vi "calibrate steering.vi"(9 "Flip direction?":bool, 10 "Steer motor port":T1=1 items=["Port A", "Port B", "Port C"], 11 "NXT":T2={"error"={"status"=FALSE, "code"=0, "source"=""}, "address"="", "NXT #"=-1, "Show Error"=TRUE, "Connection"=4} {"Connection" items=["USB", "Bluetooth", "USB then Bluetooth", "Last Connection", "Preference"]}) -> (1 "Full right":i16, 2 "Full left":i16, 3 "NXT 2":T2={"error"={"status"=FALSE, "code"=0, "source"=""}, "address"="", "NXT #"=-1, "Show Error"=TRUE, "Connection"=4} caption="NXT" {"Connection" items=["USB", "Bluetooth", "USB then Bluetooth", "Last Connection", "Preference"]})   [LabVIEW 2009]
uses:
  <vilib>/NXT/Subs/LVHSConnector.ctl
  <vilib>/NXT/Block Support/NXT_OutputPort.ctl
  <vilib>/NXT/Dual Mode Library/Motors/MotorDistance_Single.vi
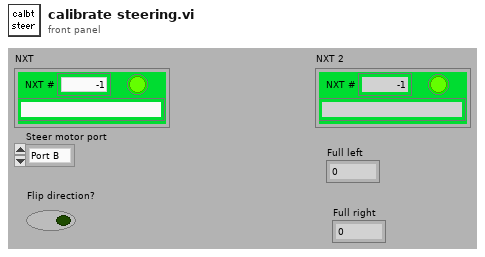
[diagram p1: front panel]
types:
  T1 = typedef "NXT_OutputPort.ctl" = u8
  T2 = typedef "LVHSConnector.ctl" = cluster{"error":errorcluster, "address":string, "NXT #":i32, "Show Error":bool, "Connection":u16}
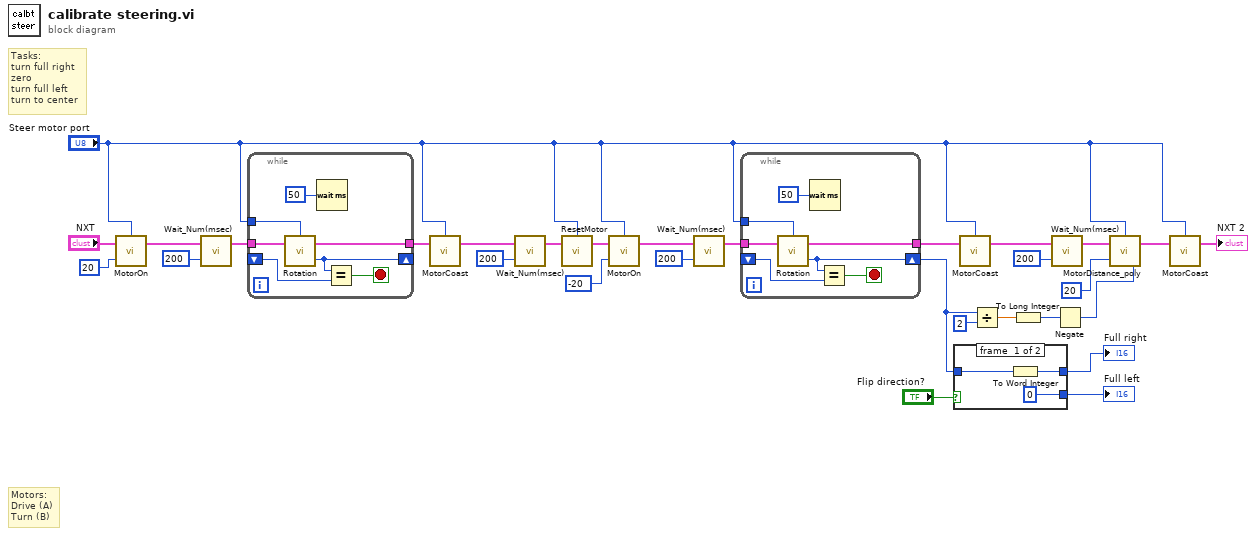
[diagram p0: block diagram]
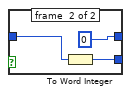
[diagram p2: hidden frame]
diagram:
  # "Motors:\nDrive (A)\nTurn (B)"
  # "Tasks:\nturn full right\nzero\nturn full left\nturn to center"
  n1 = call <vilib>:"MotorOn.vi"("Power (75)"=i8 20, "NXT"="NXT", "Output Port (All Ports)"="Steer motor port") -> ("NXT"=w6:T2)  [unwired: 1 in]
  n2 = call <vilib>:"Wait_Num(msec).vi"("Time (100 msec)"=u32 200 ("Time (msec)"), "NXT"=w6) -> ("NXT"=w5:T2)  [unwired: 2 in]
  n3 = while {
    tunnel: "Steer motor port" -> [w37]
    tunnel: w5 -> [w36]
    tunnel: [w35] -> w29
    shift-right: [w34] -> _
    shift-left: _ -> [w32]
    stop <- w33 stop-if-true
    n4 = call <vilib>:"Rotation.vi"("NXT"=w36, "Port (Port A)"=w37) -> ("Rotation"=w34:i32, "NXT"=w35:T2)  [unwired: 1 in]
    n5 = Wait (ms)(milliseconds to wait=u32 50) -> ()  [unwired: 1 out]
    n6 = Equal?(x=w34, y=w32) -> (x = y?=w33:bool)
  }
  n7 = call <vilib>:"MotorCoast.vi"("NXT"=w29, "Port (All Ports)"="Steer motor port") -> ("NXT"=w15:T2)  [unwired: 2 in]
  n8 = call <vilib>:"Wait_Num(msec).vi"("Time (100 msec)"=u32 200 ("Time (msec)"), "NXT"=w15) -> ("NXT"=w16:T2)  [unwired: 2 in]
  n9 = call <vilib>:"ResetMotor.vi"("NXT"=w16, "Port (All Ports)"="Steer motor port") -> ("NXT"=w27:T2)  [unwired: 2 in]
  n10 = call <vilib>:"MotorOn.vi"("Power (75)"=i8 -20, "NXT"=w27, "Output Port (All Ports)"="Steer motor port") -> ("NXT"=w13:T2)  [unwired: 1 in]
  n11 = call <vilib>:"Wait_Num(msec).vi"("Time (100 msec)"=u32 200 ("Time (msec)"), "NXT"=w13) -> ("NXT"=w14:T2)  [unwired: 2 in]
  n12 = while {
    tunnel: "Steer motor port" -> [w44]
    tunnel: w14 -> [w43]
    tunnel: [w42] -> w22
    shift-right: [w41] -> w3
    shift-left: _ -> [w39]
    stop <- w40 stop-if-true
    n13 = call <vilib>:"Rotation.vi"("NXT"=w43, "Port (Port A)"=w44) -> ("Rotation"=w41:i32, "NXT"=w42:T2)  [unwired: 1 in]
    n14 = Wait (ms)(milliseconds to wait=u32 50) -> ()  [unwired: 1 out]
    n15 = Equal?(x=w41, y=w39) -> (x = y?=w40:bool)
  }
  n16 = case shown="False" "Flip direction?" {
    tunnel: [i16 0 ("Full left") w49] -> w4
    tunnel: w3 -> [w46 w50]
    tunnel: [w45 i16 0 ("Full left")] -> w2
    frame #0 {
      n17 = To Word Integer(number=w46) -> (16bit integer=w45:i16)
    }
    frame #1 {
      n18 = To Word Integer(number=w50) -> (16bit integer=w49:i16)
    }
  }
  "Full left" <- w4
  "Full right" <- w2
  n19 = call <vilib>:"MotorCoast.vi"("NXT"=w22, "Port (All Ports)"="Steer motor port") -> ("NXT"=w19:T2)  [unwired: 2 in]
  n20 = Divide(x=w3, y=2) -> (x/y=w24:dbl)
  n21 = To Long Integer(number=w24) -> (32bit integer=w23:i32)
  n22 = call <vilib>:"Wait_Num(msec).vi"("Time (100 msec)"=u32 200 ("Time (msec)"), "NXT"=w19) -> ("NXT"=w18:T2)  [unwired: 2 in]
  n23 = Negate(x=w23) -> (-x=w10:i32)
  n24 = call-poly <vilib>:"MotorDistance_poly.vi"("Power (75)"=20, "Distance (100)"=w10, "NXT"=w18, "Output Port (All Ports)"="Steer motor port") -> ("NXT"=w21:T2)
  n25 = call <vilib>:"MotorCoast.vi"("NXT"=w21, "Port (All Ports)"="Steer motor port") -> ("NXT"=→"NXT 2":T2)  [unwired: 2 in]
